vi "UHR-Fleezers Control (host) - 10.5.vi"() -> ()   [LabVIEW 2011] (continued)
      tunnel: [w3324 w3335] -> w2721
      tunnel: [FALSE w3334] -> w2863
      tunnel: "Start MCL Scan" -> [_ w3329]
      tunnel: "Confocal Image" -> [_ w3328]
      tunnel: "Confocal Linescan" -> [_ _]
      frame False {
      }
      frame True {
        w3334 = TRUE
        n1728 = case shown="True" "Restart DMA? (MCL)" {
          tunnel: [w3386 w3388] -> w3339
          tunnel: [w3385 w3387] -> w3338
          tunnel: w3341 -> [w3386 w3391]
          tunnel: w3340 -> [w3385 w3390]
          frame False {
          }
          frame True {
            n1729 = call "reset FPGA DMA.vi"("error in"=w3390, "FPGA VI Reference In"=w3391) -> ("error out"=w3387:errorcluster, "FPGA VI Reference Out"=w3388:T19)
            n1730 = local write "Overflow (data lost)"(FALSE ("Overflow (data lost)")) -> ()
          }
        }
        n1731 = case shown="False" w3329 {
          selector: w3329 -> [_ w3345]
          tunnel: w3328 -> [w3344 _]
          tunnel: [w3344 w3345] -> w3327
          frame False {
            n1732 = property on="2D or 1D Scan" class="Bool (strict)"("Val(Sgnl)"=w3344) -> ()  [unwired: 2 in, 2 out]
            n1733 = property on="Confocal Image" class="Bool (strict)"("Value"=FALSE ("Start Confocal Map")) -> ()  [unwired: 2 in, 2 out]
          }
          frame True {
          }
        }
        n1734 = local write "MCL Scanning"(w3334) -> ()
        n1735 = local read "AO1"() -> (w3331:dbl)
        n1736 = local read "AO2"() -> (w3330:dbl)
        n1737 = case shown="True" "Center Scan" {
          tunnel: w3339 -> [w3352 w3384]
          tunnel: w3338 -> [w3351 w3383]
          tunnel: [w3350 w3382] -> w3336
          tunnel: [w3349 w3381] -> w3335
          tunnel: [w3347 w3368] -> w3333
          tunnel: [w3346 w3367] -> w3332
          tunnel: w3331 -> [w3347 w3373]
          tunnel: w3330 -> [w3346 w3376]
          tunnel: w3327 -> [_ _]
          frame False {
            w3348 = TRUE ("AI to FIFO")
            n1738 = xnode "Read/Write Control"("FPGA VI Reference In"=w3352, "error in"=w3351, "AI to FIFO"=w3348, "APD to FIFO"=w3348, "Start scan (MCL)"=w3348) -> ("FPGA VI Reference Out"=w3350:T19, "error out"=w3349:errorcluster)
          }
          frame True {
            w3380 = TRUE ("AI to FIFO")
            n1739 = local read "Scan steps (MCL)"() -> (w3359:u64)
            n1740 = local read "Scan lines (y)"() -> (w3355:u64)
            n1741 = local read "Fast Scan Dir"() -> (w3366:bool)
            n1742 = local read "Actual MCL Inc (V)"() -> (w3356:dbl)
            n1743 = Decrement(x=w3355) -> (x-1=w3354:u64)
            n1744 = Decrement(x=w3359) -> (x-1=w3358:u64)
            n1745 = Multiply(x=w3356, y=w3354) -> (x*y=w3353:dbl)
            n1746 = Divide(x=w3353, y=2.0) -> (x/y=w3363:dbl)
            n1747 = Multiply(x=w3356, y=w3358) -> (x*y=w3357:dbl)
            n1748 = Divide(x=w3357, y=2.0) -> (x/y=w3362:dbl)
            n1749 = Select(t=w3362, s=w3366, f=w3363) -> (s? t:f=w3361:dbl)
            n1750 = Select(t=w3363, s=w3366, f=w3362) -> (s? t:f=w3365:dbl)
            n1751 = Subtract(x=w3373, y=w3365) -> (x-y=w3364:dbl)
            n1752 = Subtract(x=w3376, y=w3361) -> (x-y=w3360:dbl)
            n1753 = local read "2D or 1D Scan"() -> (w3378:bool)
            n1754 = Not(x=w3366) -> (.not. x?=w3372:bool)
            n1755 = Not(x=w3378) -> (.not. x?=w3374:bool)
            n1756 = And(x=w3366, y=w3374) -> (x .and. y?=w3375:bool)
            n1757 = And(x=w3374, y=w3372) -> (x .and. y?=w3377:bool)
            n1758 = Select(t=w3376, s=w3377, f=w3360) -> (s? t:f=w3367:dbl)
            n1759 = Select(t=w3373, s=w3375, f=w3364) -> (s? t:f=w3368:dbl)
            n1760 = call "Volt to I16.vi"("Voltage In"=w3368) -> ("I16 Voltage Out"=w3371:i16)
            n1761 = call "Volt to I16.vi"("Voltage In"=w3367) -> ("I16 Voltage Out"=w3370:i16)
            n1762 = xnode "Read/Write Control"("FPGA VI Reference In"=w3384, "error in"=w3383, "AI to FIFO"=w3380, "APD to FIFO"=w3380, "Start scan (MCL)"=w3380, "AO1"=w3371, "AO2"=w3370) -> ("FPGA VI Reference Out"=w3382:T19, "error out"=w3381:errorcluster)
          }
        }
        "Initial Y" <- w3333
        "Initial X" <- w3332
        n1763 = local write "Tab Control 6"(T4."Imaging" ("Tab Control 6")) -> ()
        "wait to reset values" <- w3334
      }
    }
    n1764 = local read "Trap Pos Elements/DMA read"() -> (w2718:u32)
    n1765 = local read "Trap AI Elements/DMA read"() -> (w2793:u32)
    n1766 = local read "APD Elements/DMA read"() -> (w2759:u32)
    n1767 = xnode "Get APD Data"("FPGA VI Reference In"=w2722, "error in"=w2721, "Number of Elements"=w2759, "Timeout (ms)"=-1) -> ("Data"=w2758:u32[], "Elements Remaining"=→"APD FIFO Elements Remaining":u32)  [unwired: 2 out]
    n1768 = xnode "Invoke Method"("FPGA VI Reference In"=w2722, "error in"=w2721, "Number of Elements"=w2718, "Timeout (ms)"=-1) -> ("Data"=w2681:u16[], "Elements Remaining"=→"Trap Pos FIFO El Remaining":u32)  [unwired: 2 out]
    n1769 = xnode "Get Trap Data"("FPGA VI Reference In"=w2722, "error in"=w2721, "Number of Elements"=w2793, "Timeout (ms)"=-1 ("Timeout")) -> ("FPGA VI Reference Out"=w2615:T19, "error out"=w2614:errorcluster, "Data"=w2682:i16[], "Elements Remaining"=w2924:u32)
    "FIFO El. Rem." <- w2924
    n1770 = local read "Trap AI FIFO Depth"() -> (w2926:u32)
    n1771 = Subtract(x=w2926, y=w2793) -> (x-y=w2925:u32)
    n1772 = Decimate 1D Array(w2681) -> (w2678:u16[], w2680:u16[], w2679:u16[])
    n1773 = Divide(x=w2924, y=w2925) -> (x/y=w2923:dbl)
    "Buffer Status" <- w2923
    n1774 = To Unsigned Long Integer(number=w2678) -> (unsigned 32bit integer=w2677:u32[])
    n1775 = Join Numbers(hi=w2680, lo=w2679) -> ((hi.lo)=w2676:u32[])
    n1776 = Equal?(x=w2923, y=1.0) -> (x = y?=w2921:bool)
    n1777 = Join Numbers(hi=w2677, lo=w2676) -> ((hi.lo)=w2670:u64[])
    n1778 = call "IR AOM word to freq - vec.vi"("Frequency Word In (double vec)"=w2670) -> ("Frequency Out"=w2717:dbl[])
    n1779 = case "Alert buffer overflow" shown="True" w2921 {
      frame False {
      }
      frame True {
        n1780 = call <vilib>:"Beep.vi"() -> ()  [unwired: 3 in, 9 out]
        "Overflow (data lost)" <- TRUE ("Overflow (data lost)")
      }
    }
    n1781 = Decimate 1D Array(w2717) -> (w2716:dbl[], w2715:dbl[])
    n1782 = Build Array(w2716, w2715) -> (w2714:dbl[][])
    n1783 = local read "Trap Sets"() -> (w2792:u32)
    n1784 = case "Deinterlace trap data, average down PSD" shown="2" w2792 {
      tunnel: w2682 -> [w3421 w3486]
      tunnel: [w3418 w3483] -> w2785
      tunnel: [w3421 w3485] -> w2673
      tunnel: "Detector Type" -> [w3420 w3481]
      tunnel: [w3419 w3484] -> w2784
      tunnel: [w3417 w3482] -> w2898
      frame 1, Default {
        n1785 = Divide(x=w3421, y=3276.7) -> (x/y=w3422:dbl[])
        n1786 = Decimate 1D Array(w3422) -> (w3431:dbl[], w3430:dbl[], w3429:dbl[], w3428:dbl[], w3427:dbl[], w3426:dbl[], w3425:dbl[], w3424:dbl[])
        n1787 = case shown="\"IR-QPD + PSD + FB-QPD position\"" w3420 {
          tunnel: w3431 -> [w3455 w3480]
          tunnel: w3430 -> [w3454 w3479]
          tunnel: w3429 -> [w3439 w3457]
          tunnel: w3428 -> [w3440 w3467]
          tunnel: w3427 -> [w3453 w3478]
          tunnel: w3426 -> [w3452 w3477]
          tunnel: w3425 -> [w3436 w3458]
          tunnel: w3424 -> [w3435 w3456]
          tunnel: [w3434 w3464] -> w3419
          tunnel: [w3433 w3463] -> w3418
          tunnel: [w3432 w3462] -> w3417
          frame "IR-QPD + PSD + FB-QPD", Default {
            w3432 = 0  # Channel pattern
            n1788 = Divide(x=w3455, y=w3440) -> (x/y=w3442:dbl[])
            n1789 = Divide(x=w3454, y=w3440) -> (x/y=w3441:dbl[])
            n1790 = Divide(x=w3453, y=w3436) -> (x/y=w3438:dbl[])
            n1791 = Divide(x=w3452, y=w3435) -> (x/y=w3437:dbl[])
            n1792 = Build Array(w3442, w3441, w3440, w3439, w3438, w3437, w3436, w3435) -> (w3433:dbl[][])
            n1793 = Bundle("T1 Y", "T1 X", "T1 Sum", "FB Sum", "PSD Y", "PSD X", "PSD Y Sum", "PSD X Sum") -> (w3451:T40)  [unwired: 1 out]
            n1794 = Cluster To Array(cluster=w3451) -> (array=w3434:string[])
          }
          frame "IR-QPD + PSD + FB-QPD position" {
            w3462 = 3  # Channel pattern
            n1795 = Negate(x=w3458) -> (-x=w3459:dbl[])
            n1796 = Divide(x=w3480, y=w3467) -> (x/y=w3469:dbl[])
            n1797 = Divide(x=w3479, y=w3467) -> (x/y=w3468:dbl[])
            n1798 = Divide(x=w3478, y=w3458) -> (x/y=w3466:dbl[])
            n1799 = Divide(x=w3477, y=w3459) -> (x/y=w3465:dbl[])
            n1800 = Build Array(w3469, w3468, w3467, w3456, w3457, w3466, w3465, w3458) -> (w3463:dbl[][])
            n1801 = Bundle("T1 Y", "T1 X", "T1 Sum", "FB X", "FB Sum", "PSD Y", "PSD X", "PSD Y Sum") -> (w3476:T40)  [unwired: 1 out]
            n1802 = Cluster To Array(cluster=w3476) -> (array=w3464:string[])
          }
        }
      }
      frame 2 {
        n1803 = case shown="\"IR-QPD + PSD + FB-QPD X position\"" w3481 {
          tunnel: w3486 -> [w3548 w3615 w3686]
          tunnel: [w3487 w3606 w3617] -> w3485
          tunnel: [w3514 w3597 w3664] -> w3484
          tunnel: [w3513 w3560 w3631] -> w3483
          tunnel: [w3507 w3595 w3662] -> w3482
          frame "IR-QPD + PSD + FB-QPD", Default {
            w3507 = 1  # Channel pattern
            # "time average x2 the 4th signal and the 4 psd signals (detection laser)"
            # "deinterlace 3 signals from qpd"
            n1804 = Decimate 1D Array(w3548) -> (w3547:i16[], w3546:i16[], w3512:i16[], w3545:i16[], w3535:i16[], w3533:i16[], w3532:i16[], w3530:i16[])
            n1805 = Decimate 1D Array(w3512) -> (w3511:i16[], w3510:i16[])
            n1806 = Decimate 1D Array(w3547) -> (w3544:i16[], w3516:i16[])
            n1807 = Decimate 1D Array(w3546) -> (w3543:i16[], w3541:i16[])
            n1808 = Decimate 1D Array(w3545) -> (w3542:i16[], w3540:i16[])
            n1809 = call "downsample 1D array - double.vi"("Ave N"=2.0, "Array In"=w3535) -> ("Array Out"=w3534:dbl[])  [unwired: 1 out]
            n1810 = call "downsample 1D array - double.vi"("Ave N"=2.0, "Array In"=w3533) -> ("Array Out"=w3515:dbl[])  [unwired: 1 out]
            n1811 = call "downsample 1D array - double.vi"("Ave N"=2.0, "Array In"=w3532) -> ("Array Out"=w3531:dbl[])  [unwired: 1 out]
            n1812 = call "downsample 1D array - double.vi"("Ave N"=2.0, "Array In"=w3530) -> ("Array Out"=w3529:dbl[])  [unwired: 1 out]
            n1813 = Interleave 1D Arrays(w3544, w3543, w3542, w3516, w3541, w3540, w3511, w3510, w3534, w3515, w3531, w3529) -> (w3528:dbl[])
            n1814 = Divide(x=w3528, y=3276.7) -> (x/y=w3527:dbl[])
            n1815 = Decimate 1D Array(w3527) -> (w3526:dbl[], w3525:dbl[], w3524:dbl[], w3523:dbl[], w3522:dbl[], w3521:dbl[], w3509:dbl[], w3508:dbl[], w3520:dbl[], w3519:dbl[], w3518:dbl[], w3517:dbl[])
            n1816 = Divide(x=w3526, y=w3524) -> (x/y=w3494:dbl[])
            n1817 = Divide(x=w3525, y=w3524) -> (x/y=w3493:dbl[])
            n1818 = Divide(x=w3523, y=w3521) -> (x/y=w3492:dbl[])
            n1819 = Divide(x=w3522, y=w3521) -> (x/y=w3491:dbl[])
            n1820 = Divide(x=w3520, y=w3518) -> (x/y=w3490:dbl[])
            n1821 = Divide(x=w3519, y=w3517) -> (x/y=w3489:dbl[])
            n1822 = Build Array(w3494, w3493, w3524, w3492, w3491, w3521, w3509, w3508, w3490, w3489, w3518, w3517) -> (w3513:dbl[][])
            n1823 = Bundle("T1 Y", "T1 X", "T1 Sum", "T2 Y", "T2 X", "T2 Sum", "T1 FB Sum", "T2 FB Sum", "PSD Y", "PSD X", "PSD Y Sum", "PSD X Sum") -> (w3495:T41)  [unwired: 1 out]
            n1824 = To Word Integer(number=w3528) -> (16bit integer=w3487:i16[])
            n1825 = Cluster To Array(cluster=w3495) -> (array=w3514:string[])
          }
          frame "IR-QPD + PSD + FB-QPD X position" {
            w3595 = 2  # Channel pattern
            # "time average x2 the 3 psd signals (detection laser)"
            # "deinterlace 3 signals from qpds"
            n1826 = Decimate 1D Array(w3615) -> (w3614:i16[], w3613:i16[], w3596:i16[], w3612:i16[], w3558:i16[], w3555:i16[], w3552:i16[], w3583:i16[])
            n1827 = Decimate 1D Array(w3596) -> (w3581:i16[], w3579:i16[])
            n1828 = Decimate 1D Array(w3614) -> (w3611:i16[], w3598:i16[])
            n1829 = Decimate 1D Array(w3613) -> (w3610:i16[], w3608:i16[])
            n1830 = Decimate 1D Array(w3612) -> (w3609:i16[], w3607:i16[])
            n1831 = Decimate 1D Array(w3583) -> (w3582:i16[], w3580:i16[])
            n1832 = call "downsample 1D array - I16.vi"("Ave N"=2.0, "Array In"=w3558) -> ("Array Out"=w3556:i16[])  [unwired: 1 in]
            n1833 = call "downsample 1D array - I16.vi"("Ave N"=2.0, "Array In"=w3552) -> ("Array Out"=w3550:i16[])  [unwired: 1 in]
            n1834 = call "downsample 1D array - I16.vi"("Ave N"=2.0, "Array In"=w3555) -> ("Array Out"=w3553:i16[])  [unwired: 1 in]
            n1835 = Interleave 1D Arrays(w3611, w3610, w3609, w3598, w3608, w3607, w3582, w3581, w3580, w3579, w3556, w3553, w3550) -> (w3606:i16[])
            n1836 = Divide(x=w3606, y=3276.7) -> (x/y=w3605:dbl[])
            n1837 = Decimate 1D Array(w3605) -> (w3604:dbl[], w3603:dbl[], w3602:dbl[], w3601:dbl[], w3600:dbl[], w3599:dbl[], w3571:dbl[], w3569:dbl[], w3568:dbl[], w3566:dbl[], w3565:dbl[], w3564:dbl[], w3561:dbl[])
            n1838 = Negate(x=w3561) -> (-x=w3559:dbl[])
            n1839 = Divide(x=w3565, y=w3561) -> (x/y=w3563:dbl[])
            n1840 = Divide(x=w3564, y=w3559) -> (x/y=w3562:dbl[])
            n1841 = Divide(x=w3604, y=w3602) -> (x/y=w3587:dbl[])
            n1842 = Divide(x=w3603, y=w3602) -> (x/y=w3586:dbl[])
            n1843 = Divide(x=w3601, y=w3599) -> (x/y=w3585:dbl[])
            n1844 = Divide(x=w3600, y=w3599) -> (x/y=w3584:dbl[])
            n1845 = Divide(x=w3571, y=w3569) -> (x/y=w3570:dbl[])
            n1846 = Divide(x=w3568, y=w3566) -> (x/y=w3567:dbl[])
            n1847 = Build Array(w3587, w3586, w3602, w3585, w3584, w3599, w3570, w3569, w3567, w3566, w3563, w3562, w3561) -> (w3560:dbl[][])
            n1848 = Bundle("T1 Y", "T1 X", "T1 Sum", "T2 Y", "T2 X", "T2 Sum", "T1 FB X", "T1 FB Sum", "T2 FB X", "T2 FB Sum", "PSD Y", "PSD X", "PSD Y Sum") -> (w3588:T42)  [unwired: 1 out]
            n1849 = Cluster To Array(cluster=w3588) -> (array=w3597:string[])
          }
          frame "IR-QPD + PSD + FB-QPD XY positions" {
            w3662 = 4  # Channel pattern
            # "time average x2 the 3 psd signals (detection laser)"
            # "deinterlace 3 signals from qpds"
            n1850 = Decimate 1D Array(w3686) -> (w3685:i16[], w3684:i16[], w3663:i16[], w3683:i16[], w3629:i16[], w3675:i16[], w3674:i16[], w3651:i16[])
            n1851 = Decimate 1D Array "Feedback Sum"(w3663) -> (w3647:i16[], w3645:i16[])
            n1852 = Decimate 1D Array "QPD Y"(w3685) -> (w3682:i16[], w3665:i16[])
            n1853 = Decimate 1D Array "QPD X"(w3684) -> (w3681:i16[], w3679:i16[])
            n1854 = Decimate 1D Array "Feedback Y"(w3629) -> (w3628:i16[], w3627:i16[])
            n1855 = Decimate 1D Array "QPD Sum"(w3683) -> (w3680:i16[], w3678:i16[])
            n1856 = Decimate 1D Array "Feedback X"(w3651) -> (w3648:i16[], w3646:i16[])
            n1857 = call "downsample 1D array - double.vi"("Ave N"=2.0, "Array In"=w3675) -> ("Array Out"=w3650:dbl[])  [unwired: 1 out]
            n1858 = call "downsample 1D array - double.vi"("Ave N"=2.0, "Array In"=w3674) -> ("Array Out"=w3649:dbl[])  [unwired: 1 out]
            n1859 = Interleave 1D Arrays(w3682, w3681, w3680, w3665, w3679, w3678, w3628, w3648, w3647, w3627, w3646, w3645, w3650, w3649) -> (w3673:dbl[])
            n1860 = Divide(x=w3673, y=3276.7) -> (x/y=w3672:dbl[])
            n1861 = Decimate 1D Array(w3672) -> (w3671:dbl[], w3670:dbl[], w3669:dbl[], w3668:dbl[], w3667:dbl[], w3666:dbl[], w3624:dbl[], w3638:dbl[], w3622:dbl[], w3623:dbl[], w3636:dbl[], w3620:dbl[], w3634:dbl[], w3632:dbl[])
            n1862 = Negate(x=w3632) -> (-x=w3630:dbl[])
            n1863 = Divide(x=w3634, y=w3630) -> (x/y=w3633:dbl[])
            n1864 = Divide(x=w3623, y=w3620) -> (x/y=w3619:dbl[])
            n1865 = Divide(x=w3624, y=w3622) -> (x/y=w3621:dbl[])
            n1866 = Divide(x=w3671, y=w3669) -> (x/y=w3655:dbl[])
            n1867 = Divide(x=w3670, y=w3669) -> (x/y=w3654:dbl[])
            n1868 = Divide(x=w3668, y=w3666) -> (x/y=w3653:dbl[])
            n1869 = Divide(x=w3667, y=w3666) -> (x/y=w3652:dbl[])
            n1870 = Divide(x=w3638, y=w3622) -> (x/y=w3637:dbl[])
            n1871 = Divide(x=w3636, y=w3620) -> (x/y=w3635:dbl[])
            n1872 = Build Array(w3655, w3654, w3669, w3653, w3652, w3666, w3621, w3637, w3622, w3619, w3635, w3620, w3633, w3632) -> (w3631:dbl[][])
            n1873 = Bundle("T1 Y", "T1 X", "T1 Sum", "T2 Y", "T2 X", "T2 Sum", "T1 FB Y", "T1 FB X", "T1 FB Sum", "T2 FB Y", "T2 FB X", "T2 FB Sum", "PSD X", "PSD Y Sum") -> (w3618:T43)  [unwired: 1 out]
            n1874 = To Word Integer(number=w3673) -> (16bit integer=w3617:i16[])
            n1875 = Cluster To Array(cluster=w3618) -> (array=w3664:string[])
          }
        }
      }
    }
    "AI labels" <- w2784
    n1876 = Decimate 1D Array(w2758) -> (w2782:u32[], w2726:u32[])
    n1877 = local read "DMA Update Period (s)"() -> (w2794:dbl)
    n1878 = Build Array(w2782, w2726) -> (w2860:u32[][])
    n1879 = local read "Data Period (s)"() -> (w2632:dbl)
    n1880 = local read "BD 1 Frequency 2 (MHz)"() -> (w2665:dbl)
    n1881 = local read "BD 1 Frequency 1 (MHz)"() -> (w2666:dbl)
    n1882 = Decimate 1D Array(w2673) -> (w2697:i16[], w2696:i16[], w2694:i16[], w2693:i16[])  [unwired: 9 out]
    n1883 = To Double Precision Float(number=w2860) -> (double precision float=w2861:dbl[][])
    n1884 = local read "APD Integration Time (s)"() -> (w2739:dbl)
    n1885 = Multiply(x=w2632, y="Trap Pos. Disp. Downsample") -> (x*y=w2630:dbl)
    n1886 = Divide(x=w2697, y=w2696) -> (x/y=w2698:dbl[])
    n1887 = Divide(x=w2694, y=w2693) -> (x/y=w2695:dbl[])
    n1888 = feedback #4(0.0) -> (w2711:dbl)
    n1889 = Add(x=w2794, y=w2711) -> (x+y=w2900:dbl)
    n1890 = feedback-in #4(w2900) -> ()
    n1891 = local read "AOM X Cal (nm/MHz)"() -> (w2663:dbl)
    n1892 = To Time Stamp(1:w2711) -> (0:w2710:timestamp)
    n1893 = Split 1D Array(array=w2698, index="N El. to Ave.") -> (second subarray=w2701:dbl[])  [unwired: 1 out]
    n1894 = Split 1D Array(array=w2695, index="N El. to Ave.") -> (second subarray=w2700:dbl[])  [unwired: 1 out]
    n1895 = Multiply(x=w2632, y="Trap Disp. Downsample") -> (x*y=w2712:dbl)
    "Display Period (s)" <- w2712
    n1896 = for "Trap AI" {
      tunnel: [w3416] -> w2894 mode=indexing
      tunnel: w2710 -> [w3406]
      tunnel: "Trap Disp. Downsample" -> [w3414]
      tunnel: w2785 -> [w3412] mode=indexing
      tunnel: w2632 -> [w3411]
      tunnel: w2784 -> [w3410] mode=indexing
      tunnel: w2709 -> [w3409]
      tunnel: [w3408] -> w2750 mode=indexing
      tunnel: w2712 -> [w3407]
      workers-P: _ -> [_]
      n1897 = Bundle By Name("Y"=w3412, "dt"=w3411) -> (w3413:waveform(dbl))  [unwired: 1 out]
      n1898 = Set Waveform Attribute(5:w3410, 6:w3409, 7:w3413) -> (3:w3408:waveform(dbl))  [unwired: 1 in, 2 out]
      n1899 = call "downsample 1D array - double.vi"("Ave N"=w3414, "Array In"=w3412) -> ("Array Out"=w3415:dbl[])  [unwired: 1 out]
      n1900 = Bundle By Name(cluster=w3408, "t0"=w3406, "Y"=w3415, "dt"=w3407) -> (w3416:waveform(dbl))
    }
    n1901 = Bundle("BD 1 Frequency 1 (MHz)"=w2666, "BD 1 Frequency 2 (MHz)"=w2665) -> (w2667:T44)  [unwired: 1 out]
    n1902 = call <vilib>:"Mean.vi"("X"=w2700) -> ("mean"=w2688:dbl)  [unwired: 1 out]
    n1903 = call <vilib>:"Mean.vi"("X"=w2701) -> ("mean"=w2689:dbl)  [unwired: 1 out]
    n1904 = Reciprocal(x=w2712) -> (1/x=→"Trap Disp. Freq. (Hz)":dbl)
    n1905 = Cluster To Array(cluster=w2667) -> (array=w2664:dbl[])
    n1906 = local read "Trap X AI1 (DMA)"() -> (w2699:T13)
    n1907 = local read "Data points/scans (MCL)"() -> (w2872:dbl)
    n1908 = To Fixed-Point(number=w2688) -> (fixed-point=w2686:fxp<+/-,16,1>)  [unwired: 1 in]
    n1909 = To Fixed-Point(number=w2689) -> (fixed-point=w2687:fxp<+/-,16,1>)  [unwired: 1 in]
    n1910 = Bundle("Trap 1 Pos.", "Trap 2 Pos.") -> (w2708:cluster{string, string})  [unwired: 1 out]
    n1911 = Bundle By Name(cluster=w2699, "Set 1"=w2687, "Set 2"=w2686) -> (→"Trap X AI1 (DMA)":T13)
    n1912 = Cluster To Array(cluster=w2708) -> (array=w2705:string[])
    n1913 = Bundle("APD 1", "APD 2") -> (w2893:cluster{string, string})  [unwired: 1 out]
    n1914 = Select(t=-1.0, s="Negate Y Axis", f=1.0) -> (s? t:f=w2649:dbl)
    n1915 = for "Trap Position" {
      tunnel: w2714 -> [w3055] mode=indexing
      tunnel: "Trap Pos. Disp. Downsample" -> [w3054]
      tunnel: w2630 -> [w3052]
      tunnel: w2710 -> [w3051]
      tunnel: w2709 -> [w3049]
      tunnel: w2705 -> [w3048] mode=indexing
      tunnel: [w3047] -> w2619 mode=indexing
      tunnel: w2664 -> [w3045] mode=indexing
      tunnel: w2663 -> [w3043]
      tunnel: w2649 -> [w3042]
      n1916 = call "downsample 1D array - double.vi"("Ave N"=w3054, "Array In"=w3055) -> ("Array Out"=w3053:dbl[])  [unwired: 1 out]
      n1917 = Subtract(x=w3053, y=w3045) -> (x-y=w3046:dbl[])
      n1918 = Multiply(x=w3043, y=w3046) -> (x*y=w3044:dbl[])
      n1919 = Multiply(x=w3042, y=w3044) -> (x*y=w3041:dbl[])
      n1920 = Bundle By Name("Y"=w3041, "dt"=w3052, "t0"=w3051) -> (w3050:waveform(dbl))  [unwired: 1 out]
      n1921 = Set Waveform Attribute(5:w3048, 6:w3049, 7:w3050) -> (3:w3047:waveform(dbl))  [unwired: 1 in, 2 out]
    }
    n1922 = Cluster To Array(cluster=w2893) -> (array=w2890:string[])
    n1923 = for "APD" {
      tunnel: w2861 -> [w3395] mode=indexing
      tunnel: w2739 -> [w3403]
      tunnel: [w3399] -> w2746 mode=indexing
      tunnel: "APD Disp. Scale" -> [w3400]
      tunnel: w2709 -> [w3398]
      tunnel: w2890 -> [w3397] mode=indexing
      tunnel: "APD Disp. Downsample" -> [w3393]
      tunnel: [w3396] -> w2889
      workers-P: _ -> [_]
      tunnel: w2710 -> [w3392]
      n1924 = call "integrate 1D array interval - double.vi"("Ave N"=w3393, "Array In"=w3395) -> ("Array Out"=w3394:dbl[])  [unwired: 1 out]
      n1925 = Multiply(x=w3403, y=w3393) -> (x*y=w3396:dbl)
      n1926 = Divide(x=w3394, y=w3400) -> (x/y=w3401:dbl[])
      n1927 = Bundle By Name("t0"=w3392, "Y"=w3401, "dt"=w3396) -> (w3402:waveform(dbl))  [unwired: 1 out]
      n1928 = Set Waveform Attribute(5:w3397, 6:w3398, 7:w3402) -> (3:w3399:waveform(dbl))  [unwired: 1 in, 2 out]
    }
    "APD Display Period (s)" <- w2889
    n1929 = Reciprocal(x=w2889) -> (1/x=→"APD Display Freq. (Hz)":dbl)
    n1930 = local read "Display Period (s)"() -> (w2770:dbl)
    n1931 = Increment(x=w2872) -> (x+1=w2873:dbl)
    n1932 = To Double Precision Float(number=w2782) -> (double precision float=w2781:dbl[])
    n1933 = Index Array(array=w2619, index=0) -> (element=w2623:waveform(dbl))
    n1934 = Index Array(array=w2619, index=1) -> (element=w2618:waveform(dbl))
    n1935 = feedback #5(w2873) -> (w2876:dbl)
    n1936 = Select(t=0, s=w2863, f=w2876) -> (s? t:f=w2869:dbl)
    n1937 = Array Size(array=w2781) -> (size(s)=w2875:i32)
    n1938 = Add(x=w2875, y=w2869) -> (x+y=w2870:dbl)
    n1939 = Unbundle By Name(w2623) -> ("Y"=w2624:dbl[])
    n1940 = feedback #6(w2782) -> (w2859:u32[])
    n1941 = Build Array (concatenate)(w2859, w2782) -> (w2856:u32[])
    n1942 = feedback #7(w2726) -> (w2745:u32[])
    n1943 = Divide(x="Bead Sep. Int. Time (s)", y=w2770) -> (x/y=w2659:dbl)
    n1944 = Build Array (concatenate)(w2745, w2726) -> (w2744:u32[])
    n1945 = Add(x=w2624, y="FB Trap Pos Offset") -> (x+y=w2622:dbl[])
    "T1 x pos data" <- w2622
    n1946 = Greater?(x=w2870, y=w2872) -> (0:w2871:bool)
    n1947 = feedback #8(w2622) -> (w2661:dbl[])
    n1948 = Build Array (concatenate)(w2622, w2661) -> (w2660:dbl[])
    n1949 = Bundle By Name(cluster=w2623, "Y"=w2622) -> (w2621:waveform(dbl))
    n1950 = Select(t=w2869, s=w2871, f=w2870) -> (s? t:f=w2868:dbl)
    n1951 = feedback-in #5(w2868) -> ()
    n1952 = Array Size(array=w2856) -> (size(s)=w2853:i32)
    n1953 = Array Size(array=w2782) -> (size(s)=w2855:i32)
    n1954 = local read "MCL Scanning"() -> (w2866:bool)
    n1955 = local read "APD Integration Time (s)"() -> (w2753:dbl)
    n1956 = Bundle(w2621, w2618) -> (w2617:cluster{waveform(dbl), waveform(dbl)})  [unwired: 1 out]
    n1957 = Build Array (concatenate)(w2746, w2894) -> (w2748:waveform(dbl)[])
    "All Signals" <- w2748
    n1958 = Split 1D Array(array=w2660, index=w2659) -> (first subarray=w2653:dbl[])  [unwired: 1 out]
    n1959 = feedback-in #8(w2653) -> ()
    n1960 = Multiply(x=w2855, y="APD Ave N") -> (x*y=w2854:dbl)
    n1961 = Greater?(x=w2853, y=w2854) -> (0:w2857:bool)
    n1962 = Not(x=w2871) -> (.not. x?=w2865:bool)
    n1963 = Cluster To Array(cluster=w2617) -> (array=→"Trap Positions":waveform(dbl)[])
    n1964 = To Double Precision Float(number=w2726) -> (double precision float=w2725:dbl[])
    n1965 = call <vilib>:"Mean.vi"("X"=w2653) -> ("mean"=w2652:dbl)  [unwired: 1 out]
    "Mean T1 Position (nm)" <- w2652
    n1966 = Subtract(x=w2653, y=w2652) -> (x-y=w2658:dbl[])
    n1967 = Square(x=w2658) -> (x^2=w2657:dbl[])
    n1968 = And(x=w2865, y=w2866) -> (x .and. y?=w2867:bool)
    n1969 = call <vilib>:"Mean.vi"("X"=w2657) -> ("mean"=w2656:dbl)  [unwired: 1 out]
    n1970 = case shown="True" w2857 {
      tunnel: w2856 -> [w3175 w3182]
      tunnel: [w3175 w3180] -> w2799
      tunnel: w2854 -> [_ w3177]
      tunnel: w2853 -> [_ w3181]
      tunnel: w2744 -> [w3174 w3179]
      tunnel: [w3174 w3176] -> w2741
      frame False {
      }
      frame True {
        n1971 = Subtract(x=w3181, y=w3177) -> (x-y=w3178:dbl)
        n1972 = Array Subset(array=w3182, index=w3178, length=w3177) -> (w3180:u32[])
        n1973 = Array Subset(array=w3179, index=w3178, length=w3177) -> (w3176:u32[])
      }
    }
    n1974 = feedback-in #6(w2799) -> ()
    n1975 = feedback-in #7(w2741) -> ()
    n1976 = Square Root(x=w2656) -> (sqrt(x)=w2655:dbl)
    n1977 = Or(x=w2867, y=w2863) -> (x .or. y?=w2864:bool)
    n1978 = Equal?(x="Tab Control 6", y=T34."High Res Display") -> (x = y?=w2788:bool)
    n1979 = Multiply(x="APD Disp. Scale", y=w2746) -> (x*y=w2755:waveform(dbl)[])
    n1980 = Multiply(x=10.0, y=w2655) -> (x*y=→"Trap 1 Position RMS (A)":dbl)
    n1981 = Multiply(x="APD Disp. Downsample", y=w2753) -> (x*y=w2751:dbl)
    n1982 = Divide(x=w2755, y=w2751) -> (x/y=w2723:waveform(dbl)[])
    n1983 = case "For displaying the high resolution display (no downsampling)" shown="True" w2788 {
      tunnel: w2750 -> [_ w3075]
      frame False {
      }
      frame True {
        n1984 = Index Array(array=w3075, index="High Res. Display") -> (element=w3076:waveform(dbl))
        n1985 = call <vilib>:"Std Deviation and Variance.vi"("X"=w3076) -> ("mean"=w3083:dbl, "standard deviation"=w3088:dbl)  [unwired: 1 in, 1 out]
        "Mean Intensity" <- w3083
        "Sigma" <- w3088
        n1986 = Subtract(x=w3076, y=w3083) -> (x-y=w3082:waveform(dbl))
        n1987 = Select(t=w3082, s="Subtract mean", f=w3076) -> (s? t:f=→"1 Channel":waveform(dbl))
        n1988 = Divide(x=w3088, y=w3083) -> (x/y=→"Sigma/Mean":dbl)
        n1989 = feedback #9(1) -> (w3077:i32)
        n1990 = Greater Or Equal?(x=w3077, y="Slow mean N ave.") -> (x >= y?=w3090:bool)
        n1991 = Increment(x=w3077) -> (x+1=w3092:i32)
        n1992 = Select(t=1, s=w3090, f=w3092) -> (s? t:f=w3079:i32)
        n1993 = feedback-in #9(w3079) -> ()
        n1994 = feedback #10() -> (w3080:waveform(dbl))  [unwired: 1 out]
        n1995 = case shown="Default" w3077 {
          tunnel: [w3095 w3098] -> w3081
          tunnel: w3080 -> [w3097 _]
          tunnel: w3076 -> [w3096 w3098]
          frame Default {
            n1996 = call-poly <vilib>:"Append Waveforms.vi"("waveform B"=w3096, "waveform A"=w3097) -> ("waveform out"=w3095:waveform(dbl))  [unwired: 1 in, 8 out]
          }
          frame 1 {
          }
        }
        n1997 = feedback-in #10(w3081) -> ()
        n1998 = case shown="True" w3090 {
          tunnel: w3081 -> [_ w3094]
          frame False {
          }
          frame True {
            n1999 = call <vilib>:"Mean.vi"("X"=w3094) -> ("mean"=→"Slow mean":dbl)  [unwired: 1 out]
          }
        }
      }
    }
    n2000 = Index Array(array=w2723, index=0) -> (element=w2733:waveform(dbl))
    n2001 = Index Array(array=w2723, index=1) -> (element=w2731:waveform(dbl))
    n2002 = case "For computing FFTs for display" shown="True" "Compute FFT" {
      tunnel: w2750 -> [_ w3789]
      frame False {
      }
      frame True {
        n2003 = Build Array("FFT 1 Choice 1", "FFT 1 Choice 2", "FFT 2 Choice 1", "FFT 2 Choice 2") -> (w3782:u16[])
        n2004 = Array Size(array=w3789) -> (size(s)=w3788:i32)
        n2005 = feedback-in #11(w3782) -> ()
        n2006 = feedback #11(u16[] [100, 100, 100, 100]) -> (w3783:u16[])
        n2007 = feedback-in #12("# Spectra to Ave.") -> ()
        n2008 = feedback #12("# Spectra to Ave.") -> (w3780:dbl)
        n2009 = Not Equal?(x="# Spectra to Ave.", y=w3780) -> (x != y?=w3779:bool)
        n2010 = Not Equal?(x=w3782, y=w3783) -> (x != y?=w3781:bool)
        n2011 = feedback #13(1.0) -> (w3766:dbl)
        n2012 = Compound Arithmetic op=OR("Reset FFT", w3781, w3779) -> (w3764:bool)
        n2013 = Select(t=1.0, s=w3764, f=w3766) -> (s? t:f=w3768:dbl)
        n2014 = Greater?(x=w3768, y="# Spectra to Ave.") -> (0:w3787:bool)
        n2015 = Increment(x=w3768) -> (x+1=w3767:dbl)
        n2016 = feedback-in #13(w3767) -> ()
        n2017 = local read "DMA Update Period (s)"() -> (w3762:dbl)
        n2018 = Multiply(x="# Spectra to Ave.", y=w3762) -> (x*y=→"Ave. Time (s)":dbl)
        n2019 = Build Array(cluster{"f0":dbl, "df":dbl, "magnitude":dbl[]} {"f0"=0.0, "df"=0.0, "magnitude"=[]} ("PSD")) -> (w3771:cluster{"f0":dbl, "df":dbl, "magnitude":dbl[]}[])
        n2020 = Build Array(w3771, w3771, w3771, w3771) -> (w3773:T45)
        n2021 = feedback #14(w3773) -> (w3778:T45)
        n2022 = for {
          N: 4 -> [_]
          tunnel: w3782 -> [w3811] mode=indexing
          tunnel: w3789 -> [w3812]
          tunnel: w3788 -> [w3814]
          tunnel: w3764 -> [w3807]
          tunnel: w3787 -> [w3806]
          tunnel: "# Spectra to Ave." -> [w3805]
          tunnel: [w3804] -> w3777 mode=indexing
          tunnel: w3778 -> [w3809] mode=indexing
          tunnel: [w3808] -> w3765 mode=indexing
          tunnel: w3768 -> [w3803]
          n2023 = Less?(x=w3811, y=w3814) -> (x < y?=w3813:bool)
          n2024 = Index Array(array=w3812, index=w3811) -> (element=w3810:waveform(dbl))
          n2025 = case shown="True" w3813 {
            tunnel: w3810 -> [_ w3831]
            tunnel: w3809 -> [w3816 w3829]
            tunnel: [w3816 w3817] -> w3808
            tunnel: w3807 -> [_ w3828]
            tunnel: w3806 -> [_ w3821]
            tunnel: w3805 -> [_ w3820]
            tunnel: [cluster{"f0":dbl, "df":dbl, "magnitude":dbl[]} {"f0"=0.0, "df"=0.0, "magnitude"=[]} ("PSD") w3822] -> w3804
            tunnel: w3803 -> [_ w3819]
            frame False {
            }
            frame True {
              n2026 = call <vilib>:"Std Deviation and Variance.vi"("X"=w3831) -> ("mean"=w3832:dbl)  [unwired: 1 in, 2 out]
              n2027 = Subtract(x=w3831, y=w3832) -> (x-y=w3830:waveform(dbl))
              n2028 = xnode "Spectral Measurements"("Signals"=w3830) -> ("PSD"=w3824:cluster{"f0":dbl, "df":dbl, "magnitude":dbl[]})  [unwired: 1 in, 1 out]
              n2029 = case shown="False" w3828 {
                tunnel: w3829 -> [w3841 _]
                tunnel: [w3837 w3846] -> w3817
                tunnel: w3824 -> [w3840 w3847]
                tunnel: w3821 -> [w3839 _]
                frame False {
                  n2030 = Build Array (concatenate)(w3841, w3840) -> (w3838:cluster{"f0":dbl, "df":dbl, "magnitude":dbl[]}[])
                  n2031 = case shown="True" w3839 {
                    tunnel: w3838 -> [w3842 w3845]
                    tunnel: [w3842 w3843] -> w3837
                    frame False {
                    }
                    frame True {
                      n2032 = Delete From Array(array=w3845, index=0) -> (array with subset deleted=w3843:cluster{"f0":dbl, "df":dbl, "magnitude":dbl[]}[])  [unwired: 1 in, 1 out]
                    }
                  }
                }
                frame True {
                  n2033 = Build Array(w3847) -> (w3846:cluster{"f0":dbl, "df":dbl, "magnitude":dbl[]}[])
                }
              }
              n2034 = for {
                tunnel: w3817 -> [w3836] mode=indexing
                tunnel: [w3835] -> w3827 mode=indexing
                workers-P: _ -> [_]
                n2035 = Unbundle By Name(w3836) -> ("magnitude"=w3835:dbl[])
              }
              n2036 = Transpose 2D Array(2D array=w3827) -> (transposed array=w3826:dbl[][])
              n2037 = for {
                tunnel: w3826 -> [w3834] mode=indexing
                tunnel: [w3833] -> w3825 mode=indexing
                workers-P: _ -> [_]
                n2038 = Add Array Elements(numeric array=w3834) -> (sum=w3833:dbl)
              }
              n2039 = Select(t=w3820, s=w3821, f=w3819) -> (s? t:f=w3818:dbl)
              n2040 = Divide(x=w3825, y=w3818) -> (x/y=w3823:dbl[])
              n2041 = Bundle By Name(cluster=w3824, "magnitude"=w3823) -> (w3822:cluster{"f0":dbl, "df":dbl, "magnitude":dbl[]})
            }
          }
        }
        n2042 = case shown="True" w3764 {
          tunnel: w3765 -> [w3796 w3802]
          tunnel: [w3796 w3797] -> w3763
          frame False {
          }
          frame True {
            n2043 = Array Subset(array=w3802, index (row)=0 ("index"), length (row)=4 ("length"), index (col)=0 ("index"), length (col)=1 ("length")) -> (w3797:T45)
          }
        }
        n2044 = feedback-in #14(w3763) -> ()
        n2045 = Split 1D Array(array=w3777, index=2) -> (first subarray=→"FFT 1":cluster{"f0":dbl, "df":dbl, "magnitude":dbl[]}[], second subarray=→"FFT 2":cluster{"f0":dbl, "df":dbl, "magnitude":dbl[]}[])
      }
    }
    n2046 = case "For plotting results of scanning MCL" shown="True" w2864 {
      tunnel: w2863 -> [_ w3215]
      tunnel: w2781 -> [_ w3311]
      tunnel: w2872 -> [_ _]
      tunnel: w2750 -> [_ w3285]
      tunnel: w2725 -> [_ w3216]
      tunnel: w2724 -> [_ w3189]
      frame False {
      }
      frame True {
        w3196 = u32 0 items=["Horizontal", "Vertical", "Central", "1st Diagonal", "2nd Diagonal"] ("Type of Symmetry")
        w3224 = u32 0 items=["Horizontal", "Vertical", "Central", "1st Diagonal", "2nd Diagonal"] ("Type of Symmetry")
        w3227 = u32 0 items=["Horizontal", "Vertical", "Central", "1st Diagonal", "2nd Diagonal"] ("Type of Symmetry")
        w3256 = u32 0 items=["Horizontal", "Vertical", "Central", "1st Diagonal", "2nd Diagonal"] ("Type of Symmetry")
        n2047 = Index Array(array=w3285, index=10) -> (element=w3291:waveform(dbl))
        n2048 = Index Array(array=w3285, index=11) -> (element=w3288:waveform(dbl))
        n2049 = local read "Cycles/step (MCL)"() -> (w3241:u64)
        n2050 = Index Array(array=w3285, index="Channel") -> (element=w3287:waveform(dbl))
        n2051 = Unbundle(w3189) -> ("New Image"=w3188:T3, "New Image"=w3187:T3, "New Image"=w3186:T3, "New Image"=w3185:T3)
        n2052 = Unbundle By Name(w3291) -> ("Y"=w3243:dbl[])
        n2053 = Unbundle By Name(w3288) -> ("Y"=w3245:dbl[])
        n2054 = Unbundle By Name(w3287) -> ("Y"=w3250:dbl[])
        n2055 = call "downsample 1D array - double.vi"("Ave N"=w3241, "Array In"=w3243) -> ("Array Out"=w3242:dbl[])  [unwired: 1 out]
        n2056 = call "downsample 1D array - double.vi"("Ave N"=w3241, "Array In"=w3245) -> ("Array Out"=w3244:dbl[])  [unwired: 1 out]
        n2057 = call "downsample 1D array - double.vi"("Ave N"=w3241, "Array In"=w3250) -> ("Array Out"=w3249:dbl[])  [unwired: 1 out]
        n2058 = feedback #15(w3311) -> (w3312:dbl[])
        n2059 = Build Array (concatenate)(w3312, w3311) -> (w3293:dbl[])
        n2060 = feedback #16(w3216) -> (w3218:dbl[])
        n2061 = Build Array (concatenate)(w3218, w3216) -> (w3217:dbl[])
        n2062 = local read "Scan steps (MCL)"() -> (w3198:u64)
        n2063 = Select(t=w3311, s=w3215, f=w3293) -> (s? t:f=w3297:dbl[])
        n2064 = feedback-in #15(w3297) -> ()
        n2065 = Select(t=w3216, s=w3215, f=w3217) -> (s? t:f=w3199:dbl[])
        n2066 = feedback-in #16(w3199) -> ()
        n2067 = local read "Scan lines (y)"() -> (w3184:u64)
        n2068 = local read "N APD Samp/step"() -> (w3200:dbl)
        n2069 = feedback #17(w3242) -> (w3299:dbl[])
        n2070 = Build Array (concatenate)(w3299, w3242) -> (w3290:dbl[])
        n2071 = feedback #18(w3249) -> (w3309:dbl[])
        n2072 = Build Array (concatenate)(w3309, w3249) -> (w3308:dbl[])
        n2073 = feedback #19(w3244) -> (w3301:dbl[])
        n2074 = Build Array (concatenate)(w3301, w3244) -> (w3302:dbl[])
        n2075 = Select(t=w3242, s=w3215, f=w3290) -> (s? t:f=w3246:dbl[])
        n2076 = feedback-in #17(w3246) -> ()
        n2077 = Select(t=w3249, s=w3215, f=w3308) -> (s? t:f=w3248:dbl[])
        n2078 = feedback-in #18(w3248) -> ()
        n2079 = Select(t=w3244, s=w3215, f=w3302) -> (s? t:f=w3247:dbl[])
        n2080 = feedback-in #19(w3247) -> ()
        n2081 = Multiply(x=w3198, y=u64 2) -> (x*y=w3183:u64)
        n2082 = call "integrate 1D array interval - double.vi"("Ave N"=w3200, "Array In"=w3199) -> ("Array Out"=w3211:dbl[])  [unwired: 1 out]
        n2083 = call "integrate 1D array interval - double.vi"("Ave N"=w3200, "Array In"=w3297) -> ("Array Out"=w3296:dbl[])  [unwired: 1 out]
        n2084 = Array Size(array=w3211) -> (size(s)=w3212:i32)
        n2085 = Array Size(array=w3296) -> (size(s)=w3298:i32)
        n2086 = Multiply(x=w3184, y=w3183) -> (x*y=w3214:u64)
        n2087 = Multiply(x=w3184, y=w3183) -> (x*y=w3306:u64)
        n2088 = call <vilib>:"Mean.vi"("X"=w3246) -> ("mean"=w3230:dbl)  [unwired: 1 out]
        n2089 = Subtract(x=w3214, y=w3212) -> (x-y=w3205:u64)
        n2090 = call <vilib>:"Mean.vi"("X"=w3248) -> ("mean"=w3235:dbl)  [unwired: 1 out]
        n2091 = call <vilib>:"Mean.vi"("X"=w3247) -> ("mean"=w3233:dbl)  [unwired: 1 out]
        n2092 = call <vilib>:"Mean.vi"("X"=w3211) -> ("mean"=w3202:dbl)  [unwired: 1 out]
        n2093 = Subtract(x=w3306, y=w3298) -> (x-y=w3240:u64)
        n2094 = call <vilib>:"Mean.vi"("X"=w3296) -> ("mean"=w3237:dbl)  [unwired: 1 out]
        n2095 = Initialize Array(1.0 ("element"), w3205) -> (w3201:dbl[])
        n2096 = Initialize Array(1.0 ("element"), w3240) -> (w3231:dbl[])
        n2097 = Multiply(x=w3201, y=w3202) -> (x*y=w3203:dbl[])
        n2098 = Multiply(x=w3231, y=w3233) -> (x*y=w3234:dbl[])
        n2099 = Multiply(x=w3231, y=w3235) -> (x*y=w3236:dbl[])
        n2100 = Multiply(x=w3231, y=w3230) -> (x*y=w3232:dbl[])
        n2101 = Multiply(x=w3231, y=w3237) -> (x*y=w3238:dbl[])
        n2102 = Build Array (concatenate)(w3246, w3232) -> (w3300:dbl[])
        n2103 = Build Array (concatenate)(w3248, w3236) -> (w3304:dbl[])
        n2104 = Build Array (concatenate)(w3247, w3234) -> (w3303:dbl[])
        n2105 = Build Array (concatenate)(w3211, w3203) -> (w3213:dbl[])
        n2106 = Build Array (concatenate)(w3296, w3238) -> (w3305:dbl[])
        n2107 = Reshape Array(w3300, w3184, w3183) -> (w3266:dbl[][])
        n2108 = Reshape Array(w3213, w3184, w3183) -> (w3209:dbl[][])
        n2109 = Reshape Array(w3304, w3184, w3183) -> (w3258:dbl[][])
        n2110 = Reshape Array(w3303, w3184, w3183) -> (w3273:dbl[][])
        n2111 = Reshape Array(w3305, w3184, w3183) -> (w3283:dbl[][])
        n2112 = Array Subset(array=w3273, index (col)=0 ("index"), length (col)=w3198) -> (w3278:dbl[][])  [unwired: 2 in]
        n2113 = Array Subset(array=w3273, index (col)=w3198) -> (w3276:dbl[][])  [unwired: 3 in]
        n2114 = Array Subset(array=w3258, index (col)=0 ("index"), length (col)=w3198) -> (w3264:dbl[][])  [unwired: 2 in]
        n2115 = Array Subset(array=w3258, index (col)=w3198) -> (w3262:dbl[][])  [unwired: 3 in]
        n2116 = Array Subset(array=w3209, index (col)=0 ("index"), length (col)=w3198) -> (w3208:dbl[][])  [unwired: 2 in]
        n2117 = Array Subset(array=w3209, index (col)=w3198) -> (w3206:dbl[][])  [unwired: 3 in]
        n2118 = Array Subset(array=w3283, index (col)=0 ("index"), length (col)=w3198) -> (w3282:dbl[][])  [unwired: 2 in]
        n2119 = Array Subset(array=w3283, index (col)=w3198) -> (w3280:dbl[][])  [unwired: 3 in]
        n2120 = Array Subset(array=w3266, index (col)=0 ("index"), length (col)=w3198) -> (w3271:dbl[][])  [unwired: 2 in]
        n2121 = Array Subset(array=w3266, index (col)=w3198) -> (w3269:dbl[][])  [unwired: 3 in]
        n2122 = for {
          tunnel: w3278 -> [w3320] mode=indexing
          tunnel: [w3319] -> w3277 mode=indexing
          workers-P: _ -> [_]
          n2123 = Reverse 1D Array(array=w3320) -> (reversed array=w3319:dbl[])
        }
        n2124 = for {
          tunnel: w3264 -> [w3316] mode=indexing
          tunnel: [w3315] -> w3263 mode=indexing
          workers-P: _ -> [_]
          n2125 = Reverse 1D Array(array=w3316) -> (reversed array=w3315:dbl[])
        }
        n2126 = for {
          tunnel: w3208 -> [w3314] mode=indexing
          tunnel: [w3313] -> w3207 mode=indexing
          workers-P: _ -> [_]
          n2127 = Reverse 1D Array(array=w3314) -> (reversed array=w3313:dbl[])
        }
        n2128 = for {
          tunnel: w3282 -> [w3322] mode=indexing
          tunnel: [w3321] -> w3281 mode=indexing
          workers-P: _ -> [_]
          n2129 = Reverse 1D Array(array=w3322) -> (reversed array=w3321:dbl[])
        }
        n2130 = for {
          tunnel: w3271 -> [w3318] mode=indexing
          tunnel: [w3317] -> w3270 mode=indexing
          workers-P: _ -> [_]
          n2131 = Reverse 1D Array(array=w3318) -> (reversed array=w3317:dbl[])
        }
        n2132 = Index Array(array=w3283, index (row)=0) -> (element=→"Waveform Graph":dbl[])  [unwired: 1 in]
        n2133 = Add(x=w3277, y=w3276) -> (x+y=w3275:dbl[][])
        n2134 = Add(x=w3263, y=w3262) -> (x+y=w3261:dbl[][])
        n2135 = Add(x=w3207, y=w3206) -> (x+y=w3191:dbl[][])
        n2136 = Add(x=w3281, y=w3280) -> (x+y=w3255:dbl[][])
        n2137 = Add(x=w3270, y=w3269) -> (x+y=w3268:dbl[][])
        n2138 = Divide(x=w3261, y=2) -> (x/y=w3259:dbl[][])
        n2139 = Divide(x=w3275, y=2) -> (x/y=w3220:dbl[][])
        n2140 = Divide(x=w3268, y=2) -> (x/y=w3222:dbl[][])
        n2141 = To Single Precision Float(number=w3255) -> (single precision float=w3254:sgl[][])
        n2142 = Transpose 2D Array(2D array=w3259) -> (transposed array=→"Data map":dbl[][])
        n2143 = To Single Precision Float(number=w3191) -> (single precision float=w3195:sgl[][])
        n2144 = To Single Precision Float(number=w3220) -> (single precision float=w3226:sgl[][])
        n2145 = To Single Precision Float(number=w3222) -> (single precision float=w3223:sgl[][])
        n2146 = call "IMAQ ArrayToImage"("Image Pixels (Float)"=w3254, "Image"=w3188) -> ("Image Out"=w3257:T3)  [unwired: 8 in, 1 out]
        n2147 = call "IMAQ ArrayToImage"("Image Pixels (Float)"=w3195, "Image"=w3187) -> ("Image Out"=w3197:T3)  [unwired: 8 in, 1 out]
        n2148 = call "IMAQ ArrayToImage"("Image Pixels (Float)"=w3226, "Image"=w3186) -> ("Image Out"=w3228:T3)  [unwired: 8 in, 1 out]
        n2149 = call "IMAQ ArrayToImage"("Image Pixels (Float)"=w3223, "Image"=w3185) -> ("Image Out"=w3225:T3)  [unwired: 8 in, 1 out]
        n2150 = call "IMAQ Symmetry"("Type of Symmetry"=w3256, "Image Src"=w3257) -> ("Image Dst Out"=w3252:T3)  [unwired: 3 in, 1 out]
        n2151 = call "IMAQ Symmetry"("Type of Symmetry"=w3196, "Image Src"=w3197) -> ("Image Dst Out"=w3193:T3)  [unwired: 3 in, 1 out]
        n2152 = call "IMAQ Symmetry"("Type of Symmetry"=w3227, "Image Src"=w3228) -> ("Image Dst Out"=→"Detection Laser X":T3)  [unwired: 3 in, 1 out]
        n2153 = call "IMAQ Symmetry"("Type of Symmetry"=w3224, "Image Src"=w3225) -> ("Image Dst Out"=→"Detection Laser Y":T3)  [unwired: 3 in, 1 out]
        n2154 = call "IMAQ Set Simple Calibration"("Calibration Axis Info"=T35 {"Origin Pixel"={"X"=0.0, "Y"=0.0}, "Angle Relative to Horizontal (deg)"=0.0, "Axis Reference"=0}, "Grid Descriptor"=T36 {"X Step"=0.3, "Y Step"=0.3, "Unit"=enum."Undefined"}, "Image"=w3252) -> ("Calibrated Image"=→"APD 1":T3)  [unwired: 7 in, 1 out]
        n2155 = call "IMAQ Set Simple Calibration"("Calibration Axis Info"=T35 {"Origin Pixel"={"X"=0.0, "Y"=0.0}, "Angle Relative to Horizontal (deg)"=0.0, "Axis Reference"=0}, "Grid Descriptor"=T36 {"X Step"=0.3, "Y Step"=0.3, "Unit"=enum."Undefined"}, "Image"=w3193) -> ("Calibrated Image"=→"APD 2":T3)  [unwired: 7 in, 1 out]
      }
    }
    n2156 = Subtract(x=w2731, y="APD 2 Offset") -> (x-y=w2728:waveform(dbl))
    n2157 = Subtract(x=w2733, y="APD 1 Offset") -> (x-y=w2729:waveform(dbl))
    n2158 = Index Array(array=w2748, index=3) -> (element=w2808:waveform(dbl))
    n2159 = Index Array(array=w2748, index=6) -> (element=w2805:waveform(dbl))
    n2160 = Build Array(w2729, w2728) -> (→"APD Chart":waveform(dbl)[])
    n2161 = Array Size(array=w2799) -> (size(s)=w2852:i32)
    n2162 = call <vilib>:"Std Deviation and Variance.vi"("X"=w2741) -> ("standard deviation"=w2740:dbl)  [unwired: 1 in, 2 out]
    n2163 = Add Array Elements(numeric array=w2741) -> (sum=w2743:u32)
    n2164 = Add Array Elements(numeric array=w2799) -> (sum=w2862:u32)
    n2165 = call <vilib>:"Std Deviation and Variance.vi"("X"=w2799) -> ("standard deviation"=w2798:dbl)  [unwired: 1 in, 2 out]
    n2166 = Divide(x="T1 offset_x (mV)", y=1000.0) -> (x/y=w2809:dbl)
    n2167 = Divide(x=w2740, y=w2739) -> (x/y=w2736:dbl)
    "Rate sigma (Hz) 2" <- w2736
    n2168 = Multiply(x=w2739, y=w2852) -> (x*y=w2742:dbl)
    "Int. Time (s)" <- w2742
    n2169 = Divide(x=w2743, y=w2742) -> (x/y=w2737:dbl)
    "APD 2 Rate (Hz)" <- w2737
    n2170 = Divide(x=w2862, y=w2742) -> (x/y=w2796:dbl)
    "APD 1 Rate (Hz)" <- w2796
    n2171 = Divide(x=w2798, y=w2739) -> (x/y=w2797:dbl)
    "Rate sigma (Hz)" <- w2797
    n2172 = Divide(x=w2736, y=w2737) -> (x/y=→"Sigma/Mean 2":dbl)
    n2173 = Divide(x=w2797, y=w2796) -> (x/y=→"Sigma/Mean":dbl)
    n2174 = feedback-in #20("Calibration") -> ()
    n2175 = feedback #20(u16 1 ("Calibration")) -> (w2829:u16)
    n2176 = Divide(x="T2 offset_x (mV)", y=1000.0) -> (x/y=w2807:dbl)
    n2177 = case shown="0, Default" "Calibration" {
      tunnel: "T1 alpha_x (nm/V)" -> [_ w3151 w3172]
      tunnel: "T1 kappa_x (pN/nm)" -> [_ _ w3162]
      tunnel: "T2 alpha_x (nm/V)" -> [_ w3150 w3170]
      tunnel: "T2 kappa_x (pN/nm)" -> [_ _ w3163]
      tunnel: w2808 -> [w3133 w3148 w3168]
      tunnel: w2805 -> [w3132 w3146 w3166]
      tunnel: [w3133 w3145 w3165] -> w2838
      tunnel: [w3132 w3144 w3164] -> w2837
      tunnel: ["T1 X (V)" ("Label.Text") "T1 X (nm)" ("Label.Text") "T1 X (pN)" ("Label.Text")] -> w2826
      tunnel: ["T2 X (V)" ("Label.Text") "T2 X (nm)" ("Label.Text") "T2 X (pN)" ("Label.Text")] -> w2825
      tunnel: ["Position (V)" ("Label.Text") "Position (nm)" ("Label.Text") "Force (pN)" ("Label.Text")] -> w2827
      tunnel: w2807 -> [_ w3136 w3155]
      tunnel: w2809 -> [_ w3139 w3157]
      tunnel: ["Mean (V)" ("Label.Text") "Mean (nm)" ("Label.Text") "Mean (pN)" ("Label.Text")] -> w2822
      tunnel: ["Difference (V)" ("Label.Text") "Difference (nm)" ("Label.Text") "Difference (pN)" ("Label.Text")] -> w2756
      frame 0, Default {
      }
      frame 1 {
        n2178 = Unbundle By Name(w3148) -> ("Y"=w3152:dbl[])
        n2179 = Unbundle By Name(w3146) -> ("Y"=w3137:dbl[])
        n2180 = Subtract(x=w3152, y=w3139) -> (x-y=w3140:dbl[])
        n2181 = Subtract(x=w3137, y=w3136) -> (x-y=w3138:dbl[])
        n2182 = Multiply(x=w3138, y=w3150) -> (x*y=w3147:dbl[])
        n2183 = Multiply(x=w3151, y=w3140) -> (x*y=w3149:dbl[])
        n2184 = Bundle By Name(cluster=w3146, "Y"=w3147) -> (w3144:waveform(dbl))
        n2185 = Bundle By Name(cluster=w3148, "Y"=w3149) -> (w3145:waveform(dbl))
      }
      frame 2 {
        n2186 = Unbundle By Name(w3168) -> ("Y"=w3173:dbl[])
        n2187 = Unbundle By Name(w3166) -> ("Y"=w3171:dbl[])
        n2188 = Subtract(x=w3171, y=w3155) -> (x-y=w3156:dbl[])
        n2189 = Subtract(x=w3173, y=w3157) -> (x-y=w3158:dbl[])
        n2190 = Compound Arithmetic op=MULTIPLY(w3156, w3170, w3163) -> (w3167:dbl[])
        n2191 = Compound Arithmetic op=MULTIPLY(w3162, w3172, w3158) -> (w3169:dbl[])
        n2192 = Bundle By Name(cluster=w3166, "Y"=w3167) -> (w3164:waveform(dbl))
        n2193 = Bundle By Name(cluster=w3168, "Y"=w3169) -> (w3165:waveform(dbl))
      }
    }
    n2194 = Not Equal?(x=w2829, y="Calibration") -> (x != y?=w2786:bool)
    n2195 = case shown="True" w2786 {
      tunnel: w2827 -> [_ w3126]
      tunnel: w2826 -> [_ w3125]
      tunnel: w2825 -> [_ w3124]
      tunnel: w2822 -> [_ w3123]
      tunnel: w2756 -> [_ w3122]
      frame False {
      }
      frame True {
        n2196 = property on="Force" class="WFChart (strict)"("YScale.NameLbl.Text"=w3126) -> ()  [unwired: 2 in, 2 out]
        n2197 = property on="T2 X" class="DigNum (strict)"("Caption.Text"=w3124) -> ()  [unwired: 2 in, 2 out]
        n2198 = property on="T1 X" class="DigNum (strict)"("Caption.Text"=w3125) -> ()  [unwired: 2 in, 2 out]
        n2199 = property on="Mean" class="DigNum (strict)"("Caption.Text"=w3123) -> ()  [unwired: 2 in, 2 out]
        n2200 = property on="Difference" class="DigNum (strict)"("Caption.Text"=w3122) -> ()  [unwired: 2 in, 2 out]
      }
    }
    n2201 = Unbundle By Name(w2808) -> ("Y"=w2811:dbl[])
    n2202 = Unbundle By Name(w2805) -> ("Y"=w2814:dbl[])
    n2203 = Subtract(x=w2811, y=w2809) -> (x-y=w2812:dbl[])
    n2204 = Subtract(x=w2814, y=w2807) -> (x-y=w2813:dbl[])
    n2205 = Multiply(x=w2813, y="T2 alpha_x (nm/V)") -> (x*y=w2597:dbl[])
    n2206 = Multiply(x="T1 alpha_x (nm/V)", y=w2812) -> (x*y=w2598:dbl[])
    n2207 = Not(x="Trap Trig. Fl.") -> (.not. x?=w2635:bool)
    n2208 = Multiply(x=w2837, y=-1.0) -> (x*y=w2816:waveform(dbl))
    n2209 = Subtract(x=w2598, y=w2597) -> (x-y=w2804:dbl[])
    n2210 = Unbundle By Name(w2837) -> ("Y"=w2775:dbl[])
    n2211 = Unbundle By Name(w2838) -> ("Y"=w2599:dbl[])
    n2212 = Negate(x=w2804) -> (-x=w2595:dbl[])
    n2213 = Build Array(w2838, w2816) -> (→"Force":waveform(dbl)[])
